vi "Send Panel Close.vi"(5 "EventFilter Reference":T1, 9 "Time":u32, 10 "VI Refnum":refnum<vi>, 11 "Message Enqueuer in":refnum<class "Message Enqueuer.lvclass">) -> (0 "error out":errorcluster, 3 "Filtered EventDataMessage":refnum<class "PanelCloseMsg.lvclass">)   [LabVIEW 2017, in "ActorEvents.lvlib" / "PanelCloseMsg.lvclass"]
doc: "<License>\nCopyright © 2017 Composed Systems, LLC | All rights reserved\nwww.composed.io\n\nAuthor: Ethan Stern <ethan.stern@composed.io>\n\nThis software is provided \"AS IS\" WITHOUT WARRANTIES, either express or implied, AND IS FOR EDUCATIONAL PURPOSES ONLY.\n</License>"
uses:
  <vilib>/gpm_packages/@cs/mva-viewable/Source/ActorEvents/IEventAggregator Messages/PanelCloseMsg/PanelCloseMsg.lvclass
  <vilib>/ActorFramework/Message Enqueuer/Message Enqueuer.lvclass
  <vilib>/gpm_packages/@cs/mva-viewable/Source/ActorEvents/IEventFilter/EventFilter Reference.ctl
  <vilib>/gpm_packages/@cs/mva-viewable/Source/ActorEvents/IEventFilter/IEventFilter.lvclass
  C:/Program Files/National Instruments/LabVIEW 2017/vi.lib/gpm_packages/@cs/mva-viewable/Source/ActorEvents/IEventAggregator Messages/EventDataMessage/EventDataMessage.lvclass
  <vilib>/ActorFramework/Message Enqueuer/Message Priority.ctl
  <vilib>/gpm_packages/@cs/mva-viewable/Source/ActorEvents/IEventAggregator Messages/PanelCloseMsg/PanelCloseMsg.lvclass/PanelCloseMsg.ctl
  <vilib>/gpm_packages/@cs/mva-viewable/Source/ActorEvents/IEventAggregator Messages/EventDataMessage/EventDataMessage.lvclass/EventDataMessage.ctl
  <vilib>/ActorFramework/Message Enqueuer/Message Enqueuer.lvclass/Message Enqueuer.ctl
  <vilib>/ActorFramework/Message Enqueuer/Enqueue.vi
  <vilib>/Utility/error.llb/Clear Errors.vi
  <vilib>/gpm_packages/@cs/mva-viewable/Source/ActorEvents/IEventAggregator Messages/EventDataMessage/EventDataMessage.lvclass
  C:/Program Files/National Instruments/LabVIEW 2017/vi.lib/ActorFramework/Message/Message.lvclass
  <vilib>/ActorFramework/Message Priority Queue/Priority Enqueue.vi
panel:
  in  "error in (no error)":errorcluster
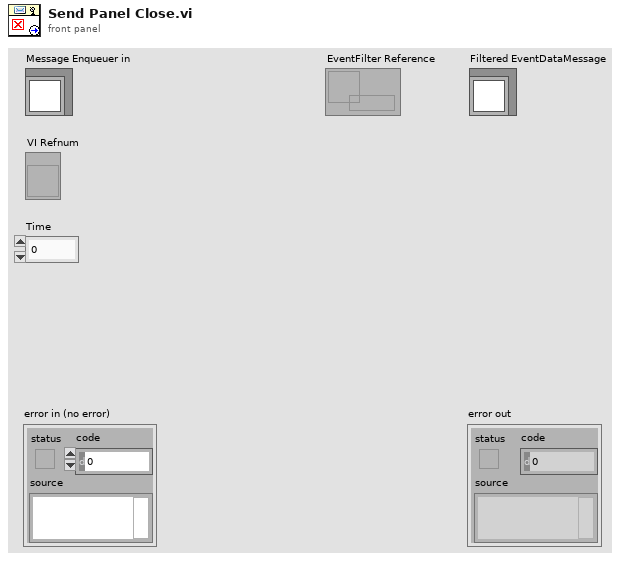
[diagram p1: front panel]
types:
  T1 = typedef "ActorEvents.lvlib/IEventFilter.lvclass/EventFilter Reference.ctl" = refnum<data-value>
  T2 = typedef "Actor Framework.lvlib/Message Enqueuer.lvclass/Message Priority.ctl" = enum16{"Low", "Normal", "High"}
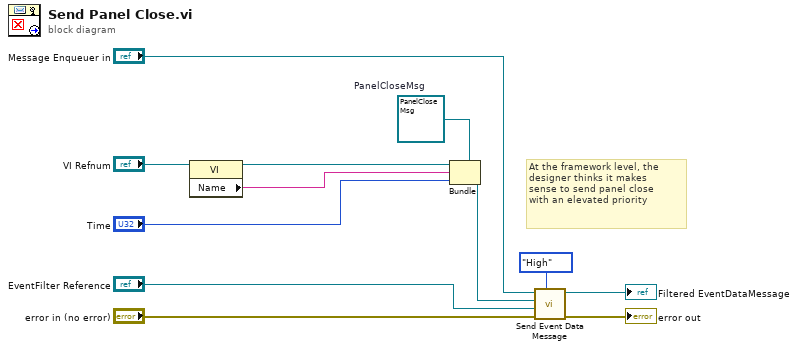
[diagram p0: block diagram]
diagram:
  w11 = refnum<class "PanelCloseMsg.lvclass"> refnum  # PanelCloseMsg
  # "At the framework level, the\ndesigner thinks it makes\nsense to send panel close\nwith an elevated priority"
  n1 = property class="VI"(reference="VI Refnum") -> (reference out=w4:refnum<vi>, "Name"=w3:string)  [unwired: 1 in, 1 out]
  n2 = Bundle(cluster=w11, w4, w3, "Time") -> (w8:refnum<class "PanelCloseMsg.lvclass">)
  n3 = call <vilib>:"Send Event Data Message.vi"("Message Priority (Normal)"=Message_Priority."High", "error in (no error)"="error in (no error)", "EventFilter Reference"="EventFilter Reference", "EventDataMessage"=w8, "Message Enqueuer in"="Message Enqueuer in") -> ("error out"=→"error out":errorcluster, "Filtered EventDataMessage"=→"Filtered EventDataMessage":refnum<class "PanelCloseMsg.lvclass">)  [unwired: 5 in]
